vi "ex3_string.vi"() -> ()   [LabVIEW 2018]
panel:
  out "String 3":string
  in  "String 2":string
  out "String":string
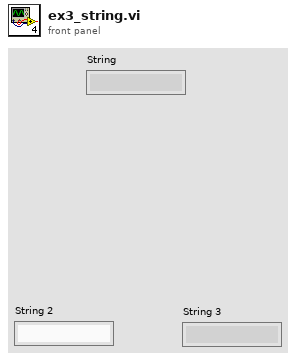
[diagram p1: front panel]
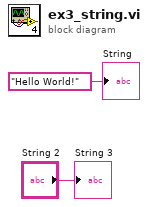
[diagram p0: block diagram]
diagram:
  "String" <- "Hello World!"
  "String 3" <- "String 2"
